vi "Serialize - Text.vi"(8 "error in (no error)":errorcluster, 11 "MC Data in":refnum<class "MC Data.lvclass">) -> (0 "error out":errorcluster, 2 "Serialized Text":string, 3 "MC Data out":refnum<class "MC Data.lvclass">)   [LabVIEW 2014, in "Alicat Lib.lvlib" / "MC Data.lvclass"]
uses:
  MC Data.lvclass
  MC Data.lvclass/MC Data.ctl
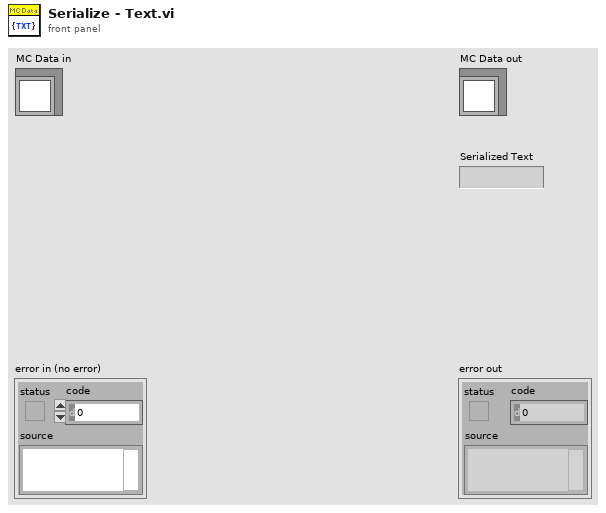
[diagram p1: front panel]
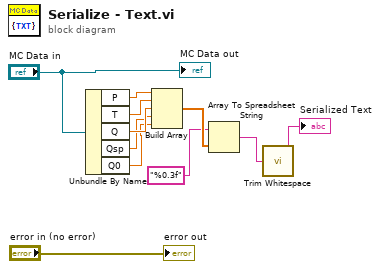
[diagram p0: block diagram]
diagram:
  n1 = Unbundle By Name("MC Data in") -> ("P"=w9:sgl, "T"=w8:sgl, "Q"=w7:sgl, "Qsp"=w6:sgl, "Q0"=w5:sgl)
  n2 = Build Array(w9, w8, w7, w6, w5) -> (w4:sgl[])
  n3 = Array To Spreadsheet String(array=w4, 3:"%0.3f" ("format string")) -> (spreadsheet string=w2:string)  [unwired: 1 in]
  n4 = call <vilib>:"Trim Whitespace.vi"("string"=w2) -> ("trimmed string"=→"Serialized Text":string)  [unwired: 1 in]
  "error out" <- "error in (no error)"
  "MC Data out" <- "MC Data in"
